vi "micron_cleanup.vi"(8 "error in":errorcluster, 10 "Micron config":T1) -> (0 "error out":errorcluster)   [LabVIEW 2014]
uses:
  micron_config.ctl
  manipulator/squiggle/Host/i2c_interface.ctl
  manipulator/squiggle/Host/fpga_reference.ctl
  testing/Micron params.ctl
  testing/stimulus.ctl
  testing/injection_point.ctl
  filtering/goal_loop_parms.ctl
  testing/mode_conrols.ctl
  testing/manipulator_cal.ctl
  asap/labview/testing/probe_calibration.ctl
  host/network_params.ctl
  cancellation/sq_control_params.ctl
  cancellation/decoupled_gain.ctl
  cancellation/estimation_controls.ctl
  asap/labview/initialization/globals.vi
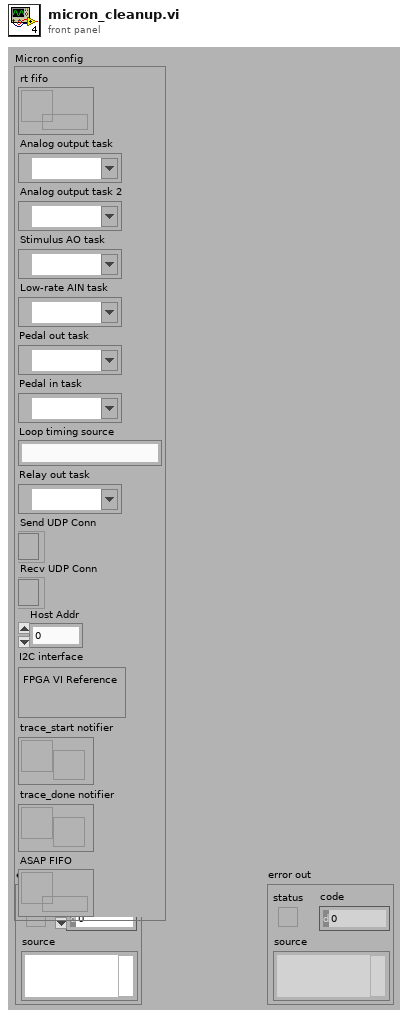
[diagram p1: front panel]
types:
  T1 = typedef "micron_config.ctl" = cluster{"rt fifo":refnum<k33>, "Analog output task":refnum<k21>, "Analog output task 2":refnum<k21>, "Stimulus AO task":refnum<k21>, "Low-rate AIN task":refnum<k21>, "Pedal out task":refnum<k21>, "Pedal in task":refnum<k21>, "Loop timing source":string, "Relay out task":refnum<k21>, "Send UDP Conn":refnum<k16>, "Recv UDP Conn":refnum<k16>, "Host Addr":u32, "I2C interface":T2, "trace_start notifier":refnum<notifier>, "trace_done notifier":refnum<notifier>, "ASAP FIFO":refnum<k33>}
  T2 = typedef "i2c_interface.ctl" = cluster{"FPGA VI Reference":T3}
  T3 = typedef "fpga_reference.ctl" = refnum<k20>
  T4 = enum16{"ASAP/Trigger", "ASAP/Finder", "ASAP/Micron", "ASAP/Micron 2", "Micron 6DOF"}
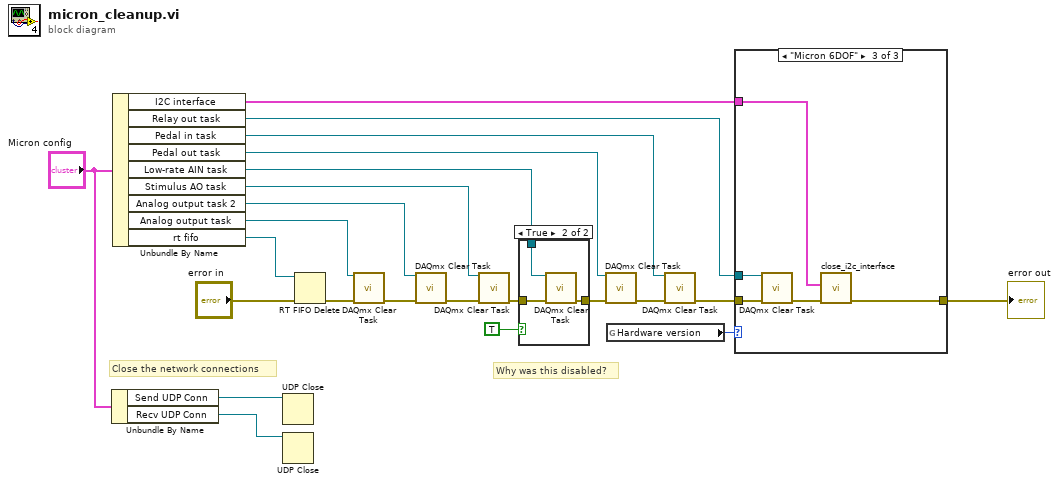
[diagram p0: block diagram]
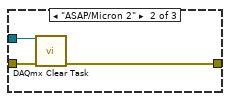
[diagram p4: hidden frame]
diagram:
  # "Why was this disabled?"
  # "Close the network connections"
  n1 = Unbundle By Name("Micron config") -> ("Send UDP Conn"=w4:refnum<k16>, "Recv UDP Conn"=w3:refnum<k16>)
  n2 = Unbundle By Name("Micron config") -> ("I2C interface"=w1:T2, "Relay out task"=w7:refnum<k21>, "Pedal in task"=w10:refnum<k21>, "Pedal out task"=w11:refnum<k21>, "Low-rate AIN task"=w17:refnum<k21>, "Stimulus AO task"=w19:refnum<k21>, "Analog output task 2"=w23:refnum<k21>, "Analog output task"=w14:refnum<k21>, "rt fifo"=w22:refnum<k33>)
  n3 = UDP Close(connection ID=w4) -> ()  [unwired: 1 in, 2 out]
  n4 = UDP Close(connection ID=w3) -> ()  [unwired: 1 in, 2 out]
  n5 = RT FIFO Delete(0:w22, 3:"error in") -> (11:w15:errorcluster)  [unwired: 1 in]
  n6 = call <vilib>:"DAQmx Clear Task.vi"("task in"=w14, "error in"=w15) -> ("error out"=w16:errorcluster)  [unwired: 13 out]
  n7 = call <vilib>:"DAQmx Clear Task.vi"("task in"=w23, "error in"=w16) -> ("error out"=w20:errorcluster)  [unwired: 13 out]
  n8 = call <vilib>:"DAQmx Clear Task.vi"("task in"=w19, "error in"=w20) -> ("error out"=w18:errorcluster)  [unwired: 13 out]
  n9 = case shown="True" TRUE {
    tunnel: w18 -> [w24 w27]
    tunnel: w17 -> [_ w26]
    tunnel: [w24 w25] -> w12
    frame False {
    }
    frame True {
      n10 = call <vilib>:"DAQmx Clear Task.vi"("task in"=w26, "error in"=w27) -> ("error out"=w25:errorcluster)  [unwired: 13 out]
    }
  }
  n11 = call <vilib>:"DAQmx Clear Task.vi"("task in"=w11, "error in"=w12) -> ("error out"=w13:errorcluster)  [unwired: 13 out]
  n12 = global read "globals.vi" "Hardware version"() -> (w9:T4)
  n13 = call <vilib>:"DAQmx Clear Task.vi"("task in"=w10, "error in"=w13) -> ("error out"=w8:errorcluster)  [unwired: 13 out]
  n14 = case shown="\"Micron 6DOF\"" w9 {
    tunnel: w8 -> [w28 w31 w36]
    tunnel: w7 -> [_ w30 w35]
    tunnel: [w28 w29 w33] -> w6
    tunnel: w1 -> [_ _ w32]
    frame "ASAP/Trigger", Default {
    }
    frame "ASAP/Micron 2" {
      n15 = call <vilib>:"DAQmx Clear Task.vi"("task in"=w30, "error in"=w31) -> ("error out"=w29:errorcluster)  [unwired: 13 out]
    }
    frame "Micron 6DOF" {
      n16 = call <vilib>:"DAQmx Clear Task.vi"("task in"=w35, "error in"=w36) -> ("error out"=w34:errorcluster)  [unwired: 13 out]
      n17 = call "close_i2c_interface.vi"("error in"=w34, "I2C interface"=w32) -> ("error out"=w33:errorcluster)  [unwired: 9 in]
    }
  }
  "error out" <- w6
